vi "poly_set_xwav_attribute_by_name.vi"(1 "value":variant, 3 "xwave in":T1={"attributes"=variant, "X"={"start"=0.0, "delta"=0.0, "units"="index", "dim"="au"}, "Y"={"data"=[], "units"="au"}}, 4 "name":string) -> (0 "xwave out":T1={"attributes"=variant, "X"={"start"=0.0, "delta"=0.0, "units"="index", "dim"="au"}, "Y"={"data"=[], "units"="au"}})   [LabVIEW 2015, in "_xwav_polys.lvlib"]
uses:
  _xwav_polys.lvlib
  xwav.ctl
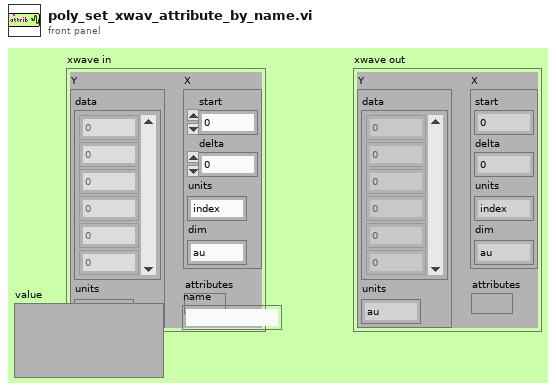
[diagram p1: front panel]
types:
  T1 = typedef "xwav.ctl" = cluster{"attributes":variant, "X":cluster{"start":dbl, "delta":dbl, "units":string, "dim":string}, "Y":cluster{"data":dbl[], "units":string}}
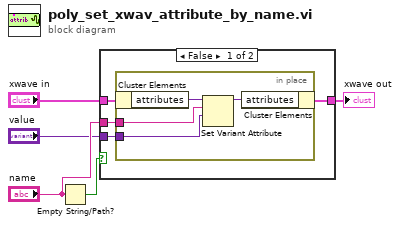
[diagram p0: block diagram]
diagram:
  n1 = Empty String/Path?(string/path="name") -> (empty?=w3:bool)
  n2 = case shown="False" w3 {
    tunnel: "xwave in" -> [w9 w14]
    tunnel: [w8 w14] -> w4
    tunnel: "name" -> [w7 _]
    tunnel: "value" -> [w6 _]
    frame False {
      n3 = in-place {
        in-place-border: w7 -> [w11]
        in-place-border: w6 -> [w10]
        n4 = in-place-cluster #1(w9) -> ("attributes"=w13:variant)
        n5 = Set Variant Attribute(Variant=w13, name=w11, value=w10) -> (Variant out=w12:variant)  [unwired: 1 in, 2 out]
        n6 = in-place-cluster #1("attributes"=w12) -> (w8:T1)
      }
    }
    frame True {
    }
  }
  "xwave out" <- w4
